vi "uart_button.vi"(0 "Data In":T5={"VESA_Staus"=enum."Init", "COM_Port"="COM35"} caption="데이터 입력", 2 "Display State In":T3 caption="디스플레이 상태 입력", 3 "Container State":T4 caption="컨테이너 상태") -> (6 "Data Out":T5={"VESA_Staus"=enum."Init", "COM_Port"="COM35"} caption="데이터 출력", 7 "Display State Out":T3 caption="디스플레이 상태 출력", 8 "Action":T2 caption="작업")   [LabVIEW 2014, in "bus_button.xctl"]
uses:
  bus_button.xctl
  data1.ctl
  VESA_Status.ctl
  <vilib>/_xctls/Container State.ctl
  Normal.ctl
  <vilib>/_xctls/Action.ctl
  SERIAL_BUTTON_PANEL.ctl
  <vilib>/Utility/sysdir.llb/System Directory Type.ctl
  <vilib>/_xctls/XControlSupport.lvlib
panel:
  in  "SERIAL":T1={"COM_Port"="COM35", "Connect"=FALSE, "Disconnect"=FALSE}
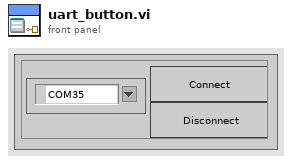
[diagram p1: front panel]
types:
  T1 = typedef "bus_button.xctl/SERIAL_BUTTON_PANEL.ctl" = cluster{"COM_Port":refnum<visa-resource-name>, "Connect":bool, "Disconnect":bool}
  T2 = typedef "XControlSupport.lvlib/Action.ctl" = cluster{"Data Changed?":bool, "State Changed?":bool, "Action Name":string}
  T3 = typedef "bus_button.xctl/Normal.ctl" = cluster{"Numeric":dbl}
  T4 = typedef "XControlSupport.lvlib/Container State.ctl" = cluster{"Indicator?":bool, "Run Mode?":bool, " Refnum":refnum<vi>}
  T5 = typedef "bus_button.xctl/data1.ctl" = cluster{"VESA_Staus":T6, "COM_Port":refnum<visa-resource-name>}
  T6 = typedef "bus_button.xctl/VESA_Status.ctl" = enum16{"Init", "Wait", "Connect", "DisConnect", "Idel", "Exit"}
  T7 = typedef "System Directory Type.ctl" = i32
  T8 = enum8{"Enabled", "Disabled", "Disabled and Grayed Out"}
  T9 = enum16{"open", "replace", "create", "open or create", "replace or create", "replace or create with confirmation"}
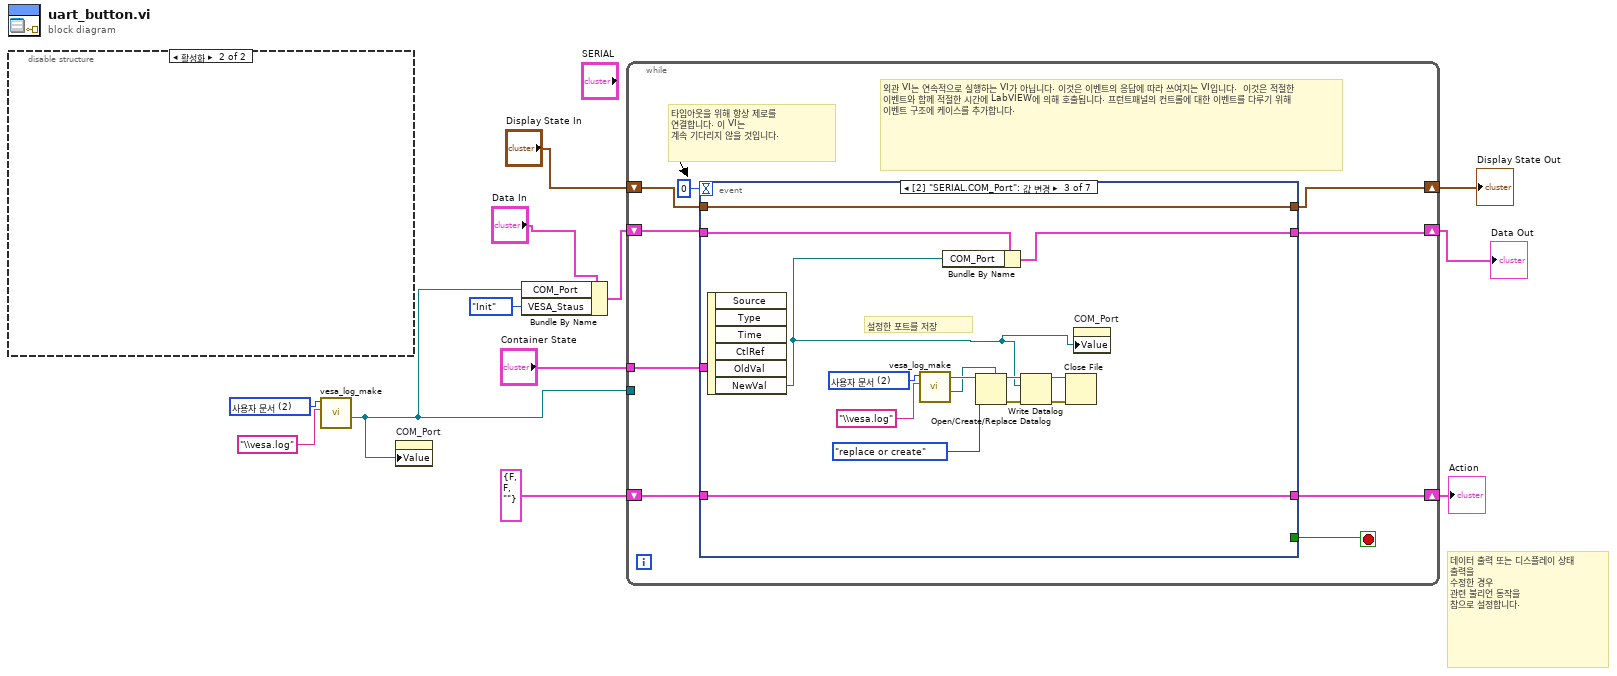
[diagram p0: block diagram]
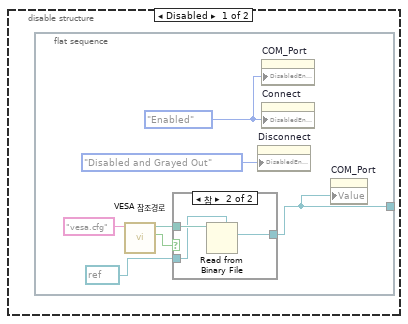
[diagram p2: hidden frame]
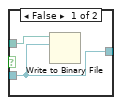
[diagram p3: hidden frame]
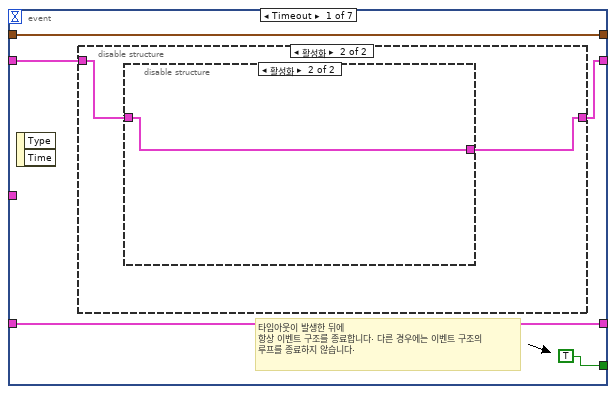
[diagram p4: hidden frame]
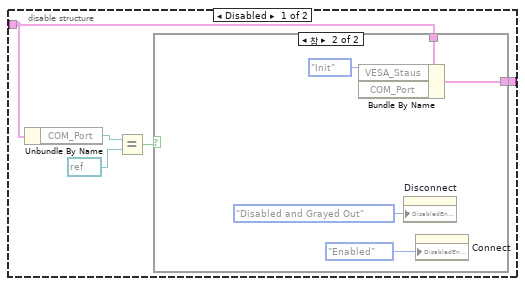
[diagram p5: hidden frame]
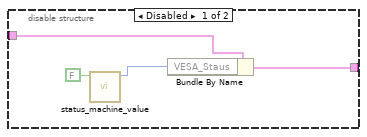
[diagram p7: hidden frame]
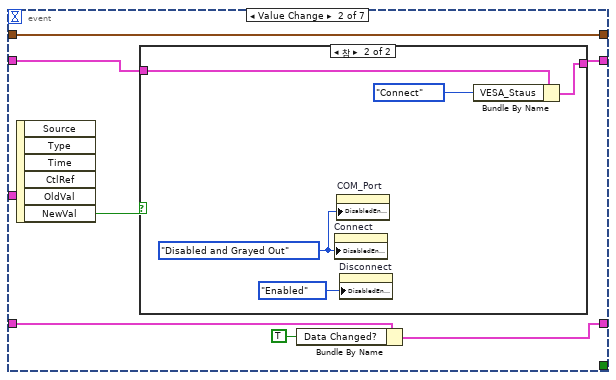
[diagram p8: hidden frame]
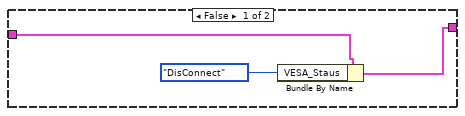
[diagram p9: hidden frame]
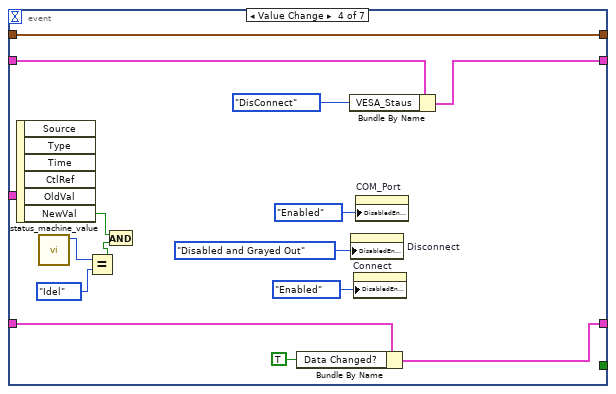
[diagram p10: hidden frame]
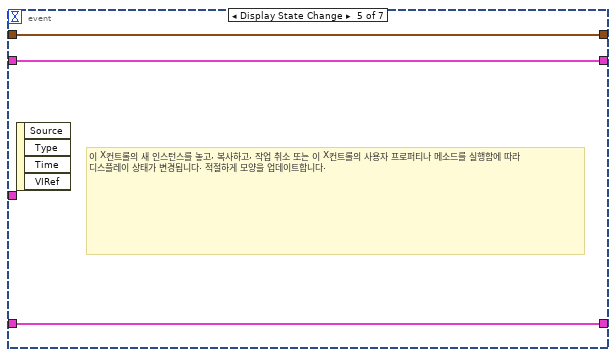
[diagram p11: hidden frame]
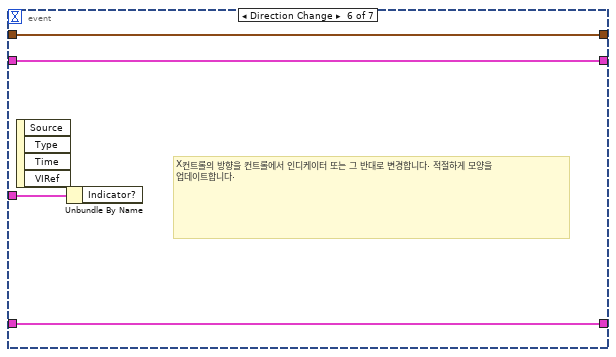
[diagram p12: hidden frame]
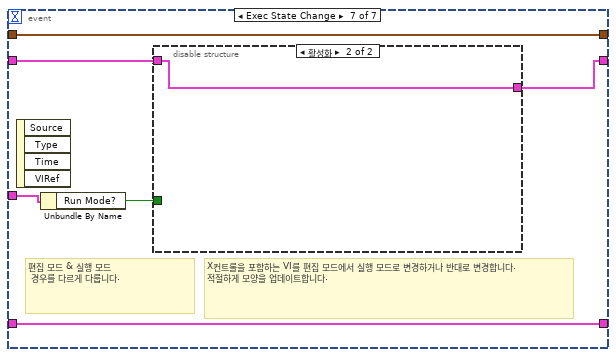
[diagram p13: hidden frame]
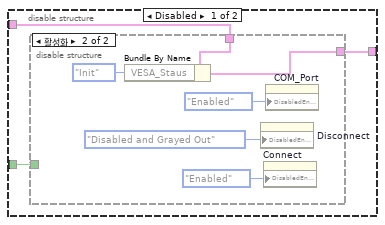
[diagram p14: hidden frame]
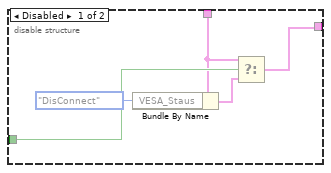
[diagram p15: hidden frame]
diagram:
  w6 = T7 2 items=["사용자 홈"=0, "사용자 데스크탑"=1, "사용자 문서"=2, "사용자 어플리케이션 데이터"=3, "사용자 환경"=4, "사용자 임시"=5, "퍼블릭 문서"=6, "퍼블릭 어플리케이션 데이터"=7, "퍼블릭 환경"=8, "퍼블릭 캐시"=13, "시스템 코어 라이브러리"=9, "시스템 설치된 라이브러리"=10, "어플리케이션 파일"=11, "부팅 볼륨 루트"=12] ("system directory type")
  # "데이터 출력 또는 디스플레이 상태 출력을\n수정한 경우\n관련 불리언 동작을\n참으로 설정합니다."
  n1 = disable-structure shown="활성화" {
    frame Disabled {
      n2 = flat-sequence {
        tunnel: [w14] -> _
        frame #0 {
          w13 = T8."Enabled" ("비활성화")
          n3 = call "VESA 참조경로.vi"("이름 또는 상대 경로"="vesa.cfg" ("File_name")) -> ("file or folder exists?"=w19:bool, "추가된 경로"=w18:path)  [unwired: 8 in, 1 out]
          n4 = case shown="참" w19 {
            tunnel: w18 -> [w21 w24]
            tunnel: [w20 w23] -> w14
            tunnel: refnum<visa-resource-name> refnum ("COM_Port") -> [w20 w22]
            frame False {
              n5 = Write to Binary File(file (use dialog)=w21, data=w20) -> ()  [unwired: 4 in, 3 out]
            }
            frame True {
              n6 = Read from Binary File(5:w22, 11:w24) -> (2:w23:refnum<visa-resource-name>)  [unwired: 4 in, 3 out]
            }
          }
          n7 = property on="Disconnect" class="Bool"("DisabledEnum"=T8."Disabled and Grayed Out" ("비활성화")) -> ()  [unwired: 2 in, 2 out]
          n8 = property on="COM_Port" class="VISAName"("DisabledEnum"=w13) -> ()  [unwired: 2 in, 2 out]
          n9 = property on="Connect" class="Bool"("DisabledEnum"=w13) -> ()  [unwired: 2 in, 2 out]
          n10 = property on="COM_Port" class="VISAName"("Value"=w14) -> ()  [unwired: 2 in, 2 out]
        }
      }
    }
    frame Enabled {
    }
  }
  n11 = call "vesa_log_make.vi"("경로와이름"="\\vesa.log", "system directory type"=w6) -> ("Serial Port"=w1:refnum<visa-resource-name>)  [unwired: 8 in, 1 out]
  n12 = property on="COM_Port" class="VISAName"("Value"=w1) -> ()  [unwired: 2 in, 2 out]
  n13 = Bundle By Name(cluster="Data In", "COM_Port"=w1, "VESA_Staus"=VESA_Status."Init") -> (w3:T5)
  n14 = while {
    shift-right: [w27] -> w8
    shift-left: T2 {"Data Changed?"=FALSE, "State Changed?"=FALSE, "Action Name"=""} ("Action") -> [w28]
    shift-right: [w32] -> w10
    shift-left: "Display State In" -> [w33]
    shift-right: [w26] -> w12
    shift-left: w3 -> [w29]
    tunnel: "Container State" -> [w30]
    tunnel: w1 -> [_]
    stop <- w31 stop-if-true
    # "외관 VI는 연속적으로 실행하는 VI가 아닙니다. 이것은 이벤트의 응답에 따라 쓰여지는 VI입니다.  이것은 적절한 이벤트와 함께 적절한 시간에 LabVIEW에 의해 호출됩니다. 프런트패널의 컨트롤에 대한 이벤트를 다루기 위해 이벤트 구조에 케이스를 추가합니다."
    # "타임아웃을 위해 항상 제로를 연결합니다. 이 VI는\n계속 기다리지 않을 것입니다."
    n15 = event shown="[2] \"SERIAL.COM_Port\": 값 변경" {
      selector: _ -> [_ _ _ _ _ _ _]
      dyn-events: _ -> [_ _ _ _ _ _ _]
      timeout: 0 -> [_ _ _ _ _ _ _]
      tunnel: w33 -> [w36 w64 w86 w100 w103 w106 w112]
      tunnel: [w36 w64 w86 w100 w103 w106 w112] -> w32
      tunnel: [TRUE _ _ _ _ _ _] -> w31
      tunnel: w30 -> [_ _ _ _ _ w107 w113]
      tunnel: w29 -> [w34 w60 w84 w96 w102 w105 w109]
      tunnel: [w35 w59 w83 w95 w102 w105 w108] -> w26
      tunnel: [w37 w62 w85 w98 w101 w104 w111] -> w27
      tunnel: w28 -> [w37 w63 w85 w99 w101 w104 w111]
      event Timeout {
        # "타임아웃이 발생한 뒤에\n항상 이벤트 구조를 종료합니다. 다른 경우에는 이벤트 구조의 루프를 종료하지 않습니다."
        n16 = event-data() -> ()  [unwired: 1 in, 2 out]
        n17 = disable-structure shown="활성화" {
          disable-tunnel: [w43 w51] -> w35
          disable-tunnel: w34 -> [w42 w52]
          frame Disabled {
            n18 = Unbundle By Name(w42) -> ("COM_Port"=w41:refnum<visa-resource-name>)
            n19 = Equal?(x=w41, y=refnum<visa-resource-name> refnum ("Serial Port")) -> (x = y?=w39:bool)
            n20 = case shown="참" w39 {
              tunnel: w42 -> [w44 w49]
              tunnel: [w44 w48] -> w43
              frame False {
              }
              frame True {
                n21 = Bundle By Name(cluster=w49, "VESA_Staus"=VESA_Status."Init") -> (w48:T5, "COM_Port"=w47:refnum<visa-resource-name>)
                n22 = property on="Disconnect" class="Bool"("DisabledEnum"=T8."Disabled and Grayed Out" ("비활성화")) -> ()  [unwired: 2 in, 2 out]
                n23 = property on="Connect" class="Bool"("DisabledEnum"=T8."Enabled" ("비활성화")) -> ()  [unwired: 2 in, 2 out]
              }
            }
          }
          frame Enabled {
            n24 = disable-structure shown="활성화" {
              disable-tunnel: w52 -> [w56 w57]
              disable-tunnel: [w54 w57] -> w51
              frame Disabled {
                n25 = call "status_machine_value.vi"("vesa상태쓰기"=FALSE) -> ("Vesa_Status"=w55:T6)  [unwired: 7 in, 3 out]
                n26 = Bundle By Name(cluster=w56, "VESA_Staus"=w55) -> (w54:T5)
              }
              frame Enabled {
              }
            }
          }
        }
      }
      event Value Change {
        n27 = event-data() -> ("NewVal"=w58:bool)  [unwired: 1 in, 5 out]
        n28 = case shown="참" w58 {
          tunnel: w60 -> [w66 w69]
          tunnel: [w65 w71] -> w59
          frame False {
            n29 = Bundle By Name(cluster=w66, "VESA_Staus"=VESA_Status."DisConnect") -> (w65:T5)
          }
          frame True {
            w70 = T8."Disabled and Grayed Out" ("비활성화")
            n30 = property on="Connect" class="Bool"("DisabledEnum"=w70) -> ()  [unwired: 2 in, 2 out]
            n31 = property on="COM_Port" class="VISAName"("DisabledEnum"=w70) -> ()  [unwired: 2 in, 2 out]
            n32 = property on="Disconnect" class="Bool"("DisabledEnum"=T8."Enabled" ("비활성화")) -> ()  [unwired: 2 in, 2 out]
            n33 = Bundle By Name(cluster=w69, "VESA_Staus"=VESA_Status."Connect") -> (w71:T5)
          }
        }
        n34 = Bundle By Name(cluster=w63, "Data Changed?"=TRUE) -> (w62:T2)
      }
      event Value Change {
        w82 = T7 2 items=["사용자 홈"=0, "사용자 데스크탑"=1, "사용자 문서"=2, "사용자 어플리케이션 데이터"=3, "사용자 환경"=4, "사용자 임시"=5, "퍼블릭 문서"=6, "퍼블릭 어플리케이션 데이터"=7, "퍼블릭 환경"=8, "퍼블릭 캐시"=13, "시스템 코어 라이브러리"=9, "시스템 설치된 라이브러리"=10, "어플리케이션 파일"=11, "부팅 볼륨 루트"=12] ("system directory type")
        # "설정한 포트를 저장"
        n35 = event-data() -> ("NewVal"=w73:refnum<visa-resource-name>)  [unwired: 1 in, 5 out]
        n36 = call "vesa_log_make.vi"("경로와이름"="\\vesa.log", "system directory type"=w82) -> ("Serial Port"=w75:refnum<visa-resource-name>, "path"=w76:path)  [unwired: 8 in]
        n37 = Bundle By Name(cluster=w84, "COM_Port"=w73) -> (w83:T5)
        n38 = Open/Create/Replace Datalog(5:w75, 10:T9."replace or create" ("동작(0:open)"), 11:w76) -> (0:w79:errorcluster, 3:w80:refnum<k1>)  [unwired: 3 in, 1 out]
        n39 = Write Datalog(4:w79, 6:w73, 7:w80) -> (0:w77:errorcluster, 3:w78:refnum<k1>)
        n40 = Close File(refnum=w78, error in=w77) -> ()  [unwired: 2 out]
        n41 = property on="COM_Port" class="VISAName"("Value"=w73) -> ()  [unwired: 2 in, 2 out]
      }
      event Value Change {
        n42 = event-data() -> ("NewVal"=w91:bool)  [unwired: 1 in, 5 out]
        n43 = call "status_machine_value.vi"() -> ("Vesa_Status"=w93:T6)  [unwired: 8 in, 3 out]
        n44 = Equal?(x=w93, y=VESA_Status."Idel" ("VESA_Staus")) -> (x = y?=w92:bool)
        n45 = And(x=w91, y=w92) -> ()  [unwired: 1 out]
        n46 = Bundle By Name(cluster=w99, "Data Changed?"=TRUE) -> (w98:T2)
        n47 = Bundle By Name(cluster=w96, "VESA_Staus"=VESA_Status."DisConnect") -> (w95:T5)
        n48 = property on="Disconnect" class="Bool"("DisabledEnum"=T8."Disabled and Grayed Out" ("비활성화")) -> ()  [unwired: 2 in, 2 out]
        n49 = property on="Connect" class="Bool"("DisabledEnum"=T8."Enabled" ("비활성화")) -> ()  [unwired: 2 in, 2 out]
        n50 = property on="COM_Port" class="VISAName"("DisabledEnum"=T8."Enabled" ("비활성화")) -> ()  [unwired: 2 in, 2 out]
      }
      event Display State Change {
        # "이 X컨트롤의 새 인스턴스를 놓고, 복사하고, 작업 취소 또는 이 X컨트롤의 사용자 프로퍼티나 메소드를 실행함에 따라 디스플레이 상태가 변경됩니다. 적절하게 모양을 업데이트합니다."
        n51 = event-data() -> ()  [unwired: 1 in, 4 out]
      }
      event Direction Change {
        # "X컨트롤의 방향을 컨트롤에서 인디케이터 또는 그 반대로 변경합니다. 적절하게 모양을 업데이트합니다."
        n52 = event-data() -> ()  [unwired: 1 in, 4 out]
        n53 = Unbundle By Name(w107) -> ()  [unwired: 1 out]
      }
      event Exec State Change {
        # "X컨트롤을 포함하는 VI를 편집 모드에서 실행 모드로 변경하거나 반대로 변경합니다.\n적절하게 모양을 업데이트합니다."
        # "편집 모드 & 실행 모드\n 경우를 다르게 다룹니다."
        n54 = event-data() -> ()  [unwired: 1 in, 4 out]
        n55 = Unbundle By Name(w113) -> ("Run Mode?"=w110:bool)
        n56 = disable-structure shown="활성화" {
          disable-tunnel: w110 -> [w116 _]
          disable-tunnel: w109 -> [w115 w128]
          disable-tunnel: [w114 w128] -> w108
          frame Disabled {
            n57 = disable-structure shown="활성화" {
              disable-tunnel: w116 -> [w121 _]
              disable-tunnel: w115 -> [w120 w124]
              disable-tunnel: [w119 w122] -> w114
              frame Disabled {
                n58 = Bundle By Name(cluster=w120, "VESA_Staus"=VESA_Status."DisConnect") -> (w118:T5)
                n59 = Select(t=w120, s=w121, f=w118) -> (s? t:f=w119:T5)
              }
              frame Enabled {
                n60 = Bundle By Name(cluster=w124, "VESA_Staus"=VESA_Status."Init") -> (w122:T5)
                n61 = property on="Disconnect" class="Bool"("DisabledEnum"=T8."Disabled and Grayed Out" ("비활성화")) -> ()  [unwired: 2 in, 2 out]
                n62 = property on="Connect" class="Bool"("DisabledEnum"=T8."Enabled" ("비활성화")) -> ()  [unwired: 2 in, 2 out]
                n63 = property on="COM_Port" class="VISAName"("DisabledEnum"=T8."Enabled" ("비활성화")) -> ()  [unwired: 2 in, 2 out]
              }
            }
          }
          frame Enabled {
          }
        }
      }
    }
  }
  "Display State Out" <- w10
  "Data Out" <- w12
  "Action" <- w8
